vi "Channel Performance Lookup Test.vi"() -> ()   [LabVIEW 2021]
uses:
  <vilib>/Platform/TimedLoop/XDataNode/timing_clust.ctl
  <vilib>/Platform/TimedLoop/XDataNode/nitl_modes.ctl
  <vilib>/Platform/TimedLoop/XDataNode/wakeup.ctl
  <vilib>/Platform/TimedLoop/XDataNode/XDataNode.xnode
  <vilib>/Platform/TimedLoop/XDataNode/XDNodeRunTimeDep.lvlib
panel:
  out "Average Empty":dbl
  out "Max Empty":dbl
  out "Avg simple string":dbl
  out "Max simple varied string":dbl
  out "Avg simple i32":dbl
  out "Max simple i32":dbl
  out "Avg simple string":dbl
  out "Max simple string":dbl
  out "pass":bool
  # "This test should be run on RT.  It stresses the communications by constantly creating resource contraints with the low priority sender and the high priority loop. On Windows the priority of the loops cannot be set."
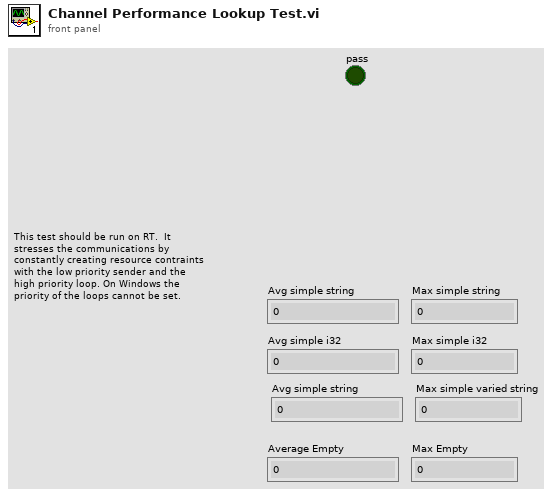
[diagram p1: front panel]
types:
  T1 = typedef "XDNodeRunTimeDep.lvlib/timing_clust.ctl" = cluster{"Expected End [f-1]":u64, "Actual End [f-1]":u64, "Finished Late? [f-1]":bool, "Expected End [i-1]":u64, "Actual End [i-1]":u64, "Finished Late? [i-1]":bool, "Expected Start [i]":u64, "Actual Start [i]":u64, "Expected Start [f]":u64, "Actual Start [f]":u64, "Source Name":string, "Structure Name":string, "Period":i64, "Deadline":i64, "Offset":i64, "Start":i64, "Priority":i32, "Timeout":i32, "Mode":T2, "Wakeup Reason":T3, "Error":errorcluster, "Source Type":string, "Secondary Source Type":string, "Global End Time":u64, "Global Start Time":u64, "Frame Duration":u64, "Iteration Duration":u64, "Assigned CPU":i32, "I/O Scan Engine Mode":u32}
  T2 = typedef "XDNodeRunTimeDep.lvlib/nitl_modes.ctl" = enum32{"No Change", "Process missed periods, maintain original phase", "Discard missed periods, maintain original phase", "Process missed periods, ignore original phase", "Discard missed periods, ignore original phase"}
  T3 = typedef "XDNodeRunTimeDep.lvlib/wakeup.ctl" = enum32{"Normal", "Aborted", "Asynchronous wakeup", "Timing source error", "Timed loop error", "Timeout"}
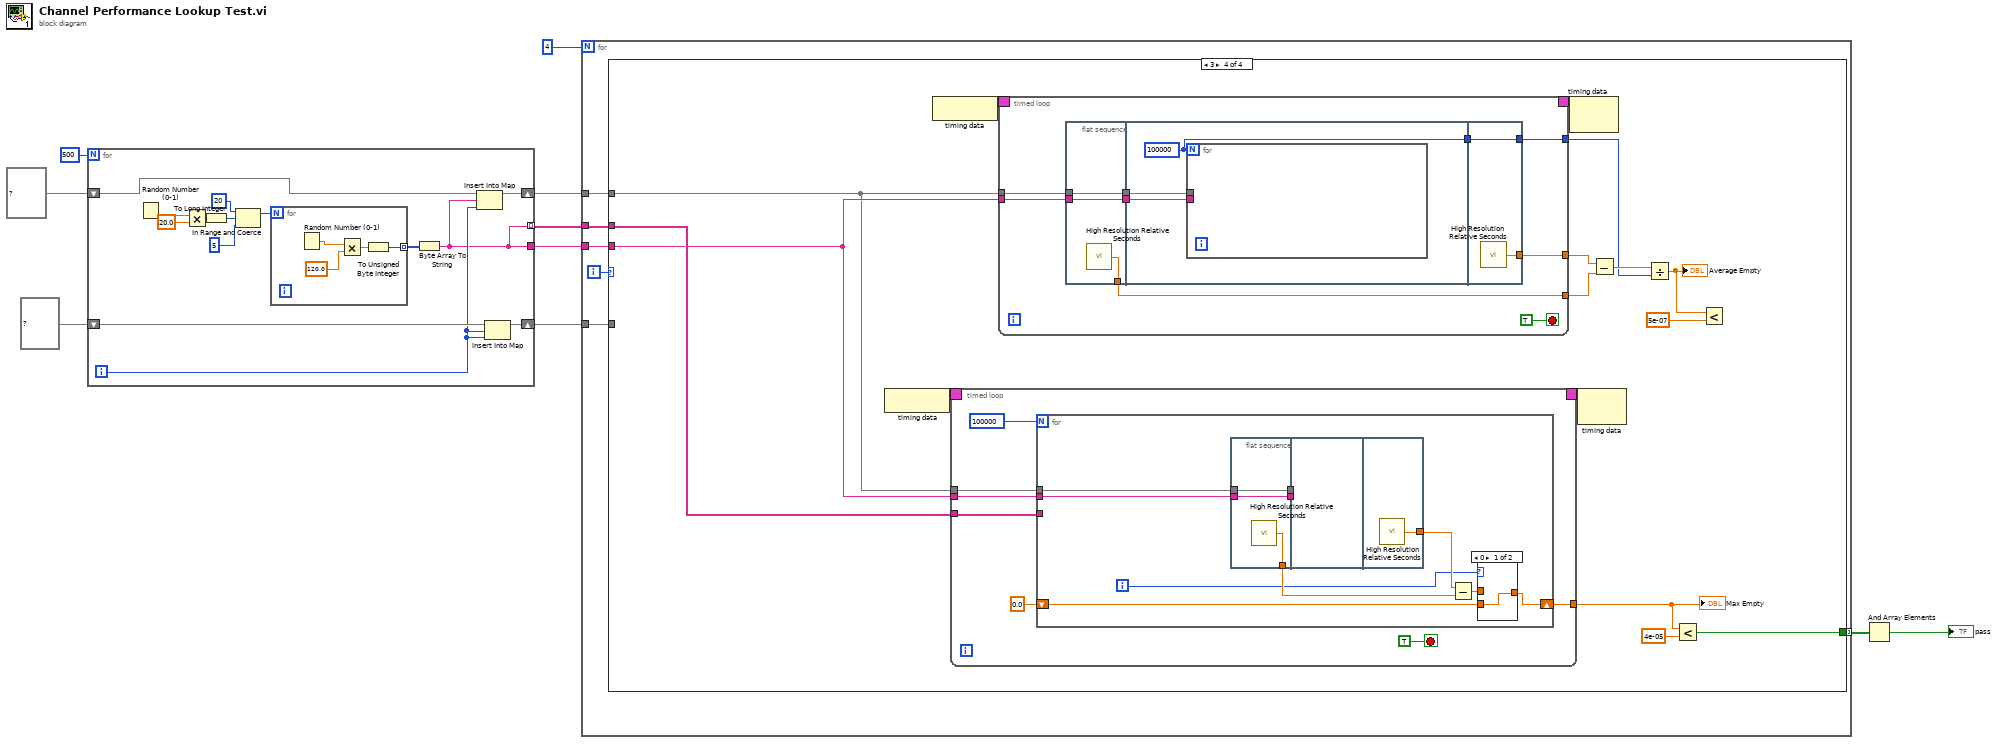
[diagram p0: block diagram]
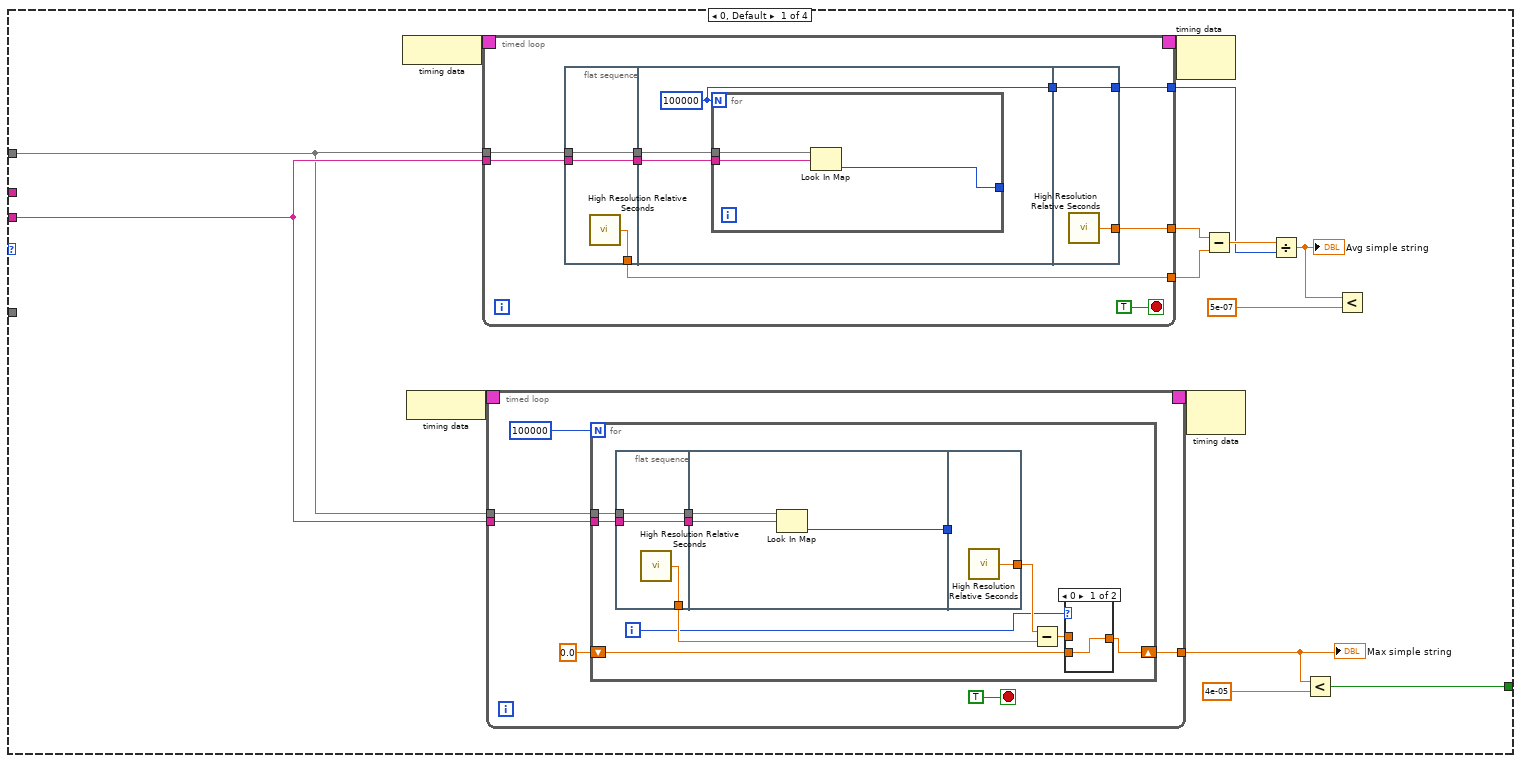
[diagram p2: hidden frame]
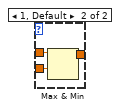
[diagram p3: hidden frame]
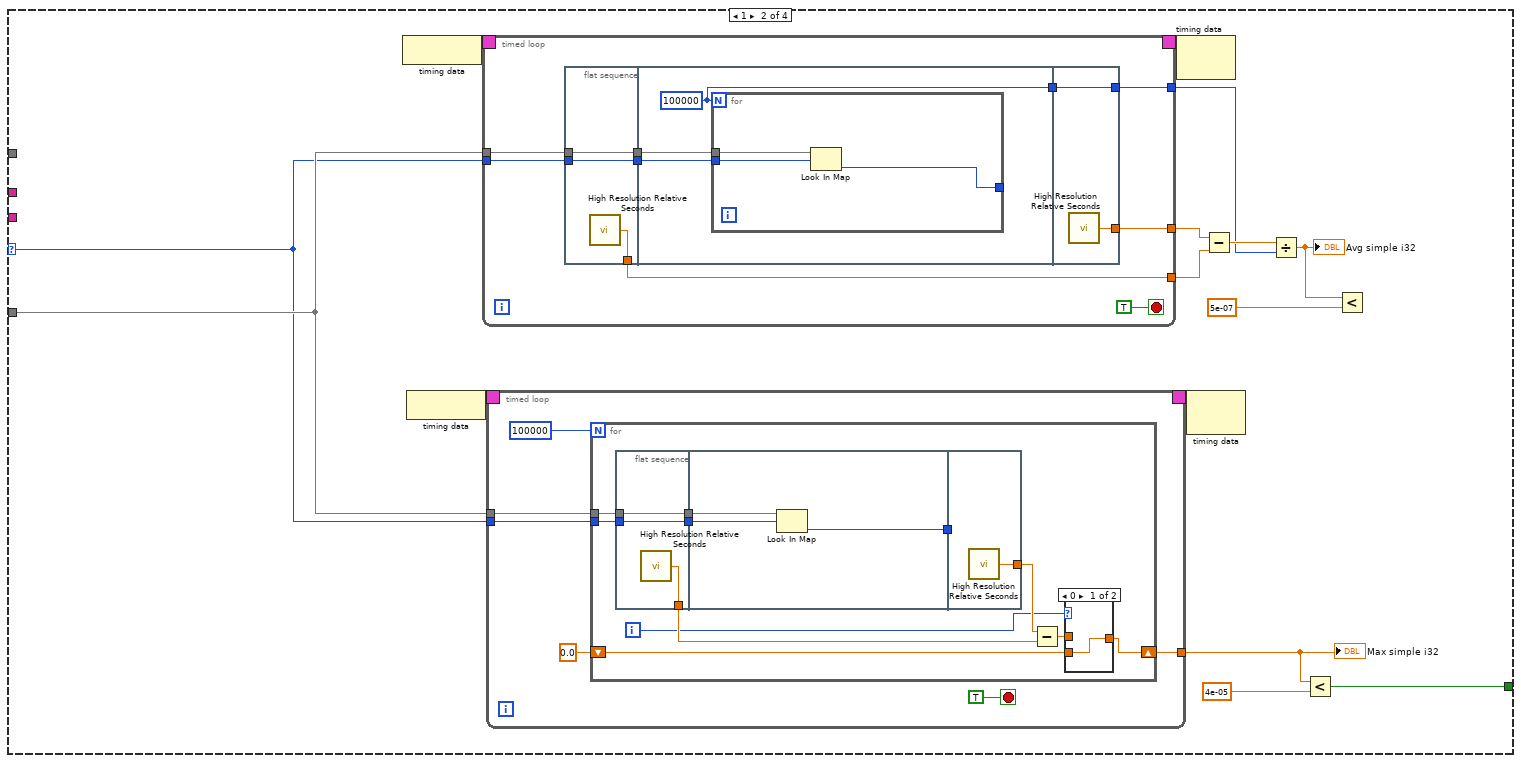
[diagram p4: hidden frame]
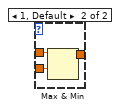
[diagram p5: hidden frame]
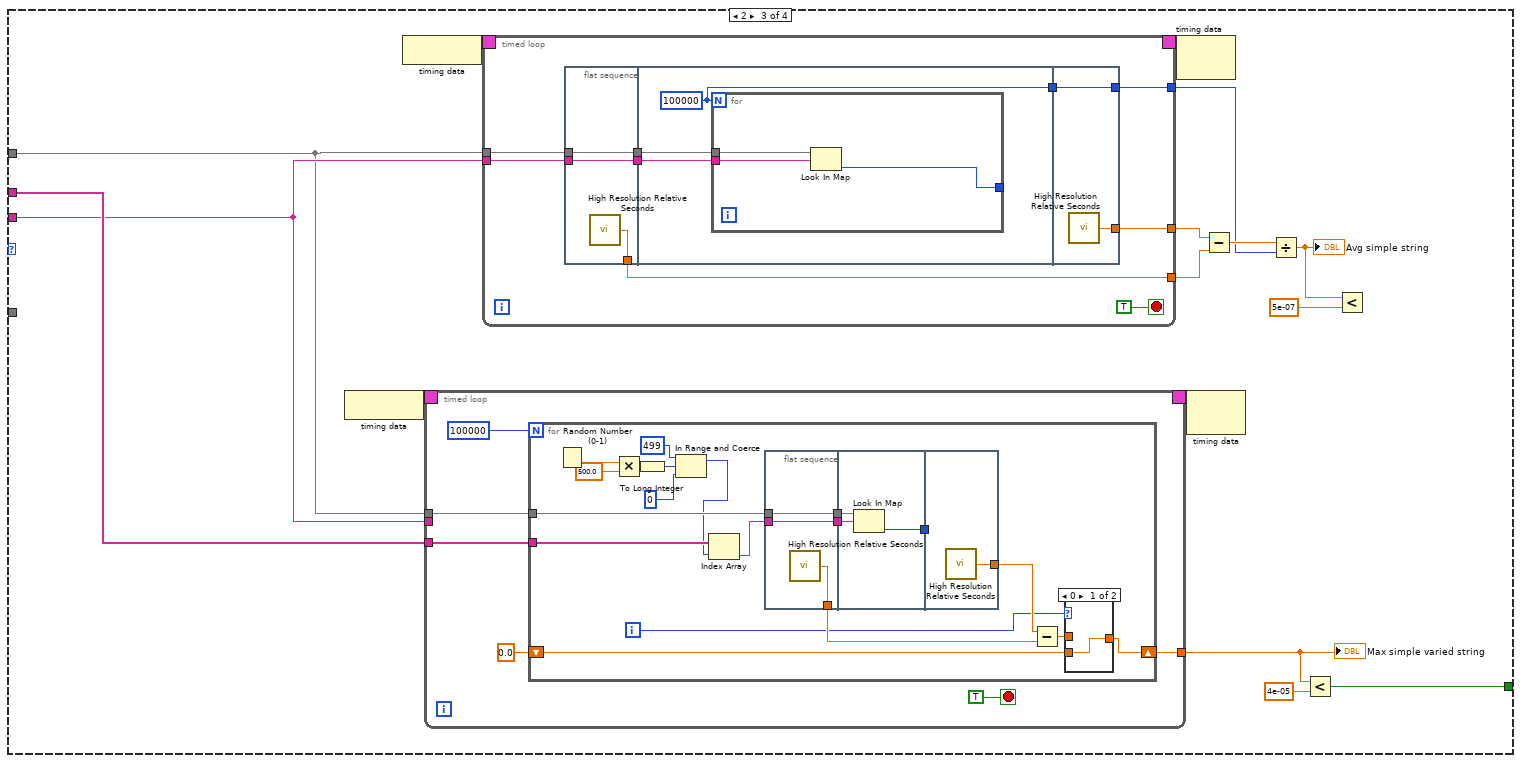
[diagram p6: hidden frame]
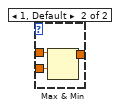
[diagram p7: hidden frame]
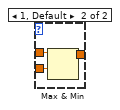
[diagram p8: hidden frame]
diagram:
  n1 = for {
    N: 500 -> [_]
    shift-right: [w16] -> w4
    shift-left: map{string, i32} {} ("map") -> [w15]
    tunnel: [w11] -> w3
    shift-right: [w13] -> w2
    shift-left: map{i32, i32} {} ("map") -> [w14]
    tunnel: [w11] -> w1 mode=indexing
    i -> [w12]
    n2 = Random Number (0-1)() -> (number: 0 to 1=w24:dbl)
    n3 = Multiply(x=w24, y=20.0) -> (x*y=w22:dbl)
    n4 = To Long Integer(number=w22) -> (32bit integer=w21:i32)
    n5 = In Range and Coerce(upper limit=20, x=w21, lower limit=5) -> (coerced(x)=w18:i32)  [unwired: 1 out]
    n6 = for {
      N: w18 -> [_]
      tunnel: [w25] -> w17 mode=indexing
      n7 = Random Number (0-1)() -> (number: 0 to 1=w28:dbl)
      n8 = Multiply(x=w28, y=120.0) -> (x*y=w26:dbl)
      n9 = To Unsigned Byte Integer(number=w26) -> (unsigned 8bit integer=w25:u8)
    }
    n10 = Byte Array To String(unsigned byte array=w17) -> (string=w11:string)
    n11 = Insert Into Map(map in=w15, key=w11, value=w12) -> (map out=w16:map{string, i32})  [unwired: 2 out]
    n12 = Insert Into Map(map in=w14, key=w12, value=w12) -> (map out=w13:map{i32, i32})  [unwired: 2 out]
  }
  n13 = for {
    N: 4 -> [_]
    tunnel: [w34] -> w9 mode=indexing
    tunnel: w4 -> [w32]
    tunnel: w3 -> [w31]
    tunnel: w2 -> [w30]
    tunnel: w1 -> [w29]
    i -> [w33]
    n14 = case shown="3" w33 {
      selector: w33 -> [_ w106 _ _]
      tunnel: [w37 w108 w180 w260] -> w34
      tunnel: w32 -> [w35 _ w177 w257]
      tunnel: w31 -> [w36 _ w178 w258]
      tunnel: w30 -> [_ w107 _ _]
      tunnel: w29 -> [_ _ w179 w259]
      frame 0, Default {
        n15 = node-c288() -> (w49:T1)
        n16 = node-c288() -> (w47:T1)
        n17 = timed-loop {
          timing: w49 -> [_]
          timing-out: [_] -> w48
          tunnel: w35 -> [w90]
          tunnel: [w87] -> w45
          tunnel: [w86] -> w44
          tunnel: [w85] -> w42
          tunnel: w36 -> [w83]
          stop <- TRUE stop-if-true
          n18 = flat-sequence {
            tunnel: w90 -> [w93]
            tunnel: [w93] -> w88
            tunnel: [w92] -> w86
            tunnel: w83 -> [w91]
            tunnel: [w91] -> w82
            tunnel: w88 -> [w96]
            tunnel: [w95] -> w84
            tunnel: w82 -> [w94]
            tunnel: [w101] -> w87
            tunnel: [w100] -> w85
            tunnel: w84 -> [w100]
            frame #0 {
              n19 = call <vilib>:"High Resolution Relative Seconds.vi"() -> ("relative seconds"=w92:dbl)
            }
            frame #1 {
              w95 = 100000
              n20 = for {
                N: w95 -> [_]
                tunnel: [w98] -> _
                tunnel: w94 -> [w97]
                tunnel: w96 -> [w99]
                n21 = Look In Map(map=w99, key=w97) -> (value=w98:i32)  [unwired: 1 in, 1 out]
              }
            }
            frame #2 {
              n22 = call <vilib>:"High Resolution Relative Seconds.vi"() -> ("relative seconds"=w101:dbl)
            }
          }
        }
        n23 = timed-loop {
          timing: w47 -> [_]
          timing-out: [_] -> w46
          tunnel: w35 -> [w51]
          tunnel: w36 -> [w50]
          tunnel: [w52] -> w39
          stop <- TRUE stop-if-true
          n24 = for {
            N: 100000 -> [_]
            shift-right: [w60] -> w52
            shift-left: 0.0 -> [w61]
            tunnel: w51 -> [w58]
            tunnel: w50 -> [w57]
            i -> [w59]
            n25 = flat-sequence {
              tunnel: [w72] -> w66
              tunnel: [w73] -> w63
              tunnel: [w71] -> w65
              tunnel: w58 -> [w72]
              tunnel: w57 -> [w71]
              tunnel: w66 -> [w76]
              tunnel: w65 -> [w75]
              tunnel: [w74] -> w56
              tunnel: [w77] -> w64
              tunnel: w56 -> [_]
              frame #0 {
                n26 = call <vilib>:"High Resolution Relative Seconds.vi"() -> ("relative seconds"=w73:dbl)
              }
              frame #1 {
                n27 = Look In Map(map=w76, key=w75) -> (value=w74:i32)  [unwired: 1 in, 1 out]
              }
              frame #2 {
                n28 = call <vilib>:"High Resolution Relative Seconds.vi"() -> ("relative seconds"=w77:dbl)
              }
            }
            n29 = Subtract(x=w64, y=w63) -> (x-y=w62:dbl)
            n30 = case shown="0" w59 {
              tunnel: w62 -> [_ w70]
              tunnel: w61 -> [w67 w69]
              tunnel: [w67 w68] -> w60
              frame 0 {
              }
              frame 1, Default {
                n31 = Max & Min(x=w70, y=w69) -> (max(x,y)=w68:dbl)  [unwired: 1 out]
              }
            }
          }
        }
        "Max simple string" <- w39
        n32 = node-c288(w48) -> ()  [unwired: 1 out]
        n33 = node-c288(w46) -> ()  [unwired: 1 out]
        n34 = Subtract(x=w45, y=w44) -> (x-y=w43:dbl)
        n35 = Divide(x=w43, y=w42) -> (x/y=w41:dbl)
        "Avg simple string" <- w41
        n36 = Less?(x=w39, y=4e-05) -> (x < y?=w37:bool)
        n37 = Less?(x=w41, y=5e-07) -> ()  [unwired: 1 out]
      }
      frame 1 {
        n38 = node-c288() -> (w120:T1)
        n39 = node-c288() -> (w118:T1)
        n40 = timed-loop {
          timing: w120 -> [_]
          timing-out: [_] -> w119
          tunnel: w107 -> [w161]
          tunnel: [w158] -> w116
          tunnel: [w157] -> w115
          tunnel: [w156] -> w113
          tunnel: w106 -> [w154]
          stop <- TRUE stop-if-true
          n41 = flat-sequence {
            tunnel: w161 -> [w164]
            tunnel: [w164] -> w159
            tunnel: [w163] -> w157
            tunnel: w154 -> [w162]
            tunnel: [w162] -> w153
            tunnel: w159 -> [w167]
            tunnel: [w166] -> w155
            tunnel: w153 -> [w165]
            tunnel: [w172] -> w158
            tunnel: [w171] -> w156
            tunnel: w155 -> [w171]
            frame #0 {
              n42 = call <vilib>:"High Resolution Relative Seconds.vi"() -> ("relative seconds"=w163:dbl)
            }
            frame #1 {
              w166 = 100000
              n43 = for {
                N: w166 -> [_]
                tunnel: [w169] -> _
                tunnel: w165 -> [w168]
                tunnel: w167 -> [w170]
                n44 = Look In Map(map=w170, key=w168) -> (value=w169:i32)  [unwired: 1 in, 1 out]
              }
            }
            frame #2 {
              n45 = call <vilib>:"High Resolution Relative Seconds.vi"() -> ("relative seconds"=w172:dbl)
            }
          }
        }
        n46 = timed-loop {
          timing: w118 -> [_]
          timing-out: [_] -> w117
          tunnel: w107 -> [w122]
          tunnel: w106 -> [w121]
          tunnel: [w123] -> w110
          stop <- TRUE stop-if-true
          n47 = for {
            N: 100000 -> [_]
            shift-right: [w131] -> w123
            shift-left: 0.0 -> [w132]
            tunnel: w122 -> [w129]
            tunnel: w121 -> [w128]
            i -> [w130]
            n48 = flat-sequence {
              tunnel: [w143] -> w137
              tunnel: [w144] -> w134
              tunnel: [w142] -> w136
              tunnel: w129 -> [w143]
              tunnel: w128 -> [w142]
              tunnel: w137 -> [w147]
              tunnel: w136 -> [w146]
              tunnel: [w145] -> w127
              tunnel: [w148] -> w135
              tunnel: w127 -> [_]
              frame #0 {
                n49 = call <vilib>:"High Resolution Relative Seconds.vi"() -> ("relative seconds"=w144:dbl)
              }
              frame #1 {
                n50 = Look In Map(map=w147, key=w146) -> (value=w145:i32)  [unwired: 1 in, 1 out]
              }
              frame #2 {
                n51 = call <vilib>:"High Resolution Relative Seconds.vi"() -> ("relative seconds"=w148:dbl)
              }
            }
            n52 = Subtract(x=w135, y=w134) -> (x-y=w133:dbl)
            n53 = case shown="0" w130 {
              tunnel: w133 -> [_ w141]
              tunnel: w132 -> [w138 w140]
              tunnel: [w138 w139] -> w131
              frame 0 {
              }
              frame 1, Default {
                n54 = Max & Min(x=w141, y=w140) -> (max(x,y)=w139:dbl)  [unwired: 1 out]
              }
            }
          }
        }
        "Max simple i32" <- w110
        n55 = node-c288(w119) -> ()  [unwired: 1 out]
        n56 = node-c288(w117) -> ()  [unwired: 1 out]
        n57 = Subtract(x=w116, y=w115) -> (x-y=w114:dbl)
        n58 = Divide(x=w114, y=w113) -> (x/y=w112:dbl)
        "Avg simple i32" <- w112
        n59 = Less?(x=w110, y=4e-05) -> (x < y?=w108:bool)
        n60 = Less?(x=w112, y=5e-07) -> ()  [unwired: 1 out]
      }
      frame 2 {
        n61 = node-c288() -> (w190:T1)
        n62 = node-c288() -> (w192:T1)
        n63 = timed-loop {
          timing: w190 -> [_]
          timing-out: [_] -> w189
          tunnel: w177 -> [w194]
          tunnel: w178 -> [_]
          tunnel: [w195] -> w182
          tunnel: w179 -> [w193]
          stop <- TRUE stop-if-true
          n64 = for {
            N: 100000 -> [_]
            shift-right: [w211] -> w195
            shift-left: 0.0 -> [w212]
            tunnel: w194 -> [w210]
            tunnel: w193 -> [w208]
            i -> [w207]
            n65 = Random Number (0-1)() -> (number: 0 to 1=w205:dbl)
            n66 = Multiply(x=w205, y=500.0) -> (x*y=w203:dbl)
            n67 = To Long Integer(number=w203) -> (32bit integer=w202:i32)
            n68 = In Range and Coerce(upper limit=499, x=w202, lower limit=0) -> (coerced(x)=w199:i32)  [unwired: 1 out]
            n69 = Index Array(array=w208, index=w199) -> (element=w206:string)
            n70 = flat-sequence {
              tunnel: [w223] -> w217
              tunnel: [w224] -> w214
              tunnel: [w222] -> w216
              tunnel: w210 -> [w223]
              tunnel: w206 -> [w222]
              tunnel: w217 -> [w227]
              tunnel: w216 -> [w226]
              tunnel: [w225] -> w209
              tunnel: [w228] -> w215
              tunnel: w209 -> [_]
              frame #0 {
                n71 = call <vilib>:"High Resolution Relative Seconds.vi"() -> ("relative seconds"=w224:dbl)
              }
              frame #1 {
                n72 = Look In Map(map=w227, key=w226) -> (value=w225:i32)  [unwired: 1 in, 1 out]
              }
              frame #2 {
                n73 = call <vilib>:"High Resolution Relative Seconds.vi"() -> ("relative seconds"=w228:dbl)
              }
            }
            n74 = Subtract(x=w215, y=w214) -> (x-y=w213:dbl)
            n75 = case shown="0" w207 {
              tunnel: w213 -> [_ w221]
              tunnel: w212 -> [w218 w220]
              tunnel: [w218 w219] -> w211
              frame 0 {
              }
              frame 1, Default {
                n76 = Max & Min(x=w221, y=w220) -> (max(x,y)=w219:dbl)  [unwired: 1 out]
              }
            }
          }
        }
        "Max simple varied string" <- w182
        n77 = timed-loop {
          timing: w192 -> [_]
          timing-out: [_] -> w191
          tunnel: w177 -> [w241]
          tunnel: [w238] -> w188
          tunnel: [w237] -> w187
          tunnel: [w236] -> w185
          tunnel: w178 -> [w234]
          stop <- TRUE stop-if-true
          n78 = flat-sequence {
            tunnel: w241 -> [w244]
            tunnel: [w244] -> w239
            tunnel: [w243] -> w237
            tunnel: w234 -> [w242]
            tunnel: [w242] -> w233
            tunnel: w239 -> [w247]
            tunnel: [w246] -> w235
            tunnel: w233 -> [w245]
            tunnel: [w252] -> w238
            tunnel: [w251] -> w236
            tunnel: w235 -> [w251]
            frame #0 {
              n79 = call <vilib>:"High Resolution Relative Seconds.vi"() -> ("relative seconds"=w243:dbl)
            }
            frame #1 {
              w246 = 100000
              n80 = for {
                N: w246 -> [_]
                tunnel: [w249] -> _
                tunnel: w245 -> [w248]
                tunnel: w247 -> [w250]
                n81 = Look In Map(map=w250, key=w248) -> (value=w249:i32)  [unwired: 1 in, 1 out]
              }
            }
            frame #2 {
              n82 = call <vilib>:"High Resolution Relative Seconds.vi"() -> ("relative seconds"=w252:dbl)
            }
          }
        }
        n83 = node-c288(w191) -> ()  [unwired: 1 out]
        n84 = node-c288(w189) -> ()  [unwired: 1 out]
        n85 = Subtract(x=w188, y=w187) -> (x-y=w186:dbl)
        n86 = Divide(x=w186, y=w185) -> (x/y=w184:dbl)
        "Avg simple string" <- w184
        n87 = Less?(x=w182, y=4e-05) -> (x < y?=w180:bool)
        n88 = Less?(x=w184, y=5e-07) -> ()  [unwired: 1 out]
      }
      frame 3 {
        n89 = node-c288() -> (w270:T1)
        n90 = node-c288() -> (w272:T1)
        n91 = timed-loop {
          timing: w270 -> [_]
          timing-out: [_] -> w269
          tunnel: w257 -> [w275]
          tunnel: w258 -> [w273]
          tunnel: [w276] -> w262
          tunnel: w259 -> [w274]
          stop <- TRUE stop-if-true
          n92 = for {
            N: 100000 -> [_]
            shift-right: [w285] -> w276
            shift-left: 0.0 -> [w286]
            tunnel: w275 -> [w282]
            tunnel: w274 -> [_]
            tunnel: w273 -> [w280]
            i -> [w284]
            n93 = flat-sequence {
              tunnel: [w296] -> w288
              tunnel: [w295] -> w283
              tunnel: w282 -> [w295]
              tunnel: [w294] -> w281
              tunnel: w280 -> [w294]
              tunnel: w283 -> [_]
              tunnel: w281 -> [_]
              tunnel: [w297] -> w289
              frame #0 {
                n94 = call <vilib>:"High Resolution Relative Seconds.vi"() -> ("relative seconds"=w296:dbl)
              }
              frame #1 {
              }
              frame #2 {
                n95 = call <vilib>:"High Resolution Relative Seconds.vi"() -> ("relative seconds"=w297:dbl)
              }
            }
            n96 = Subtract(x=w289, y=w288) -> (x-y=w287:dbl)
            n97 = case shown="0" w284 {
              tunnel: w287 -> [_ w293]
              tunnel: w286 -> [w290 w292]
              tunnel: [w290 w291] -> w285
              frame 0 {
              }
              frame 1, Default {
                n98 = Max & Min(x=w293, y=w292) -> (max(x,y)=w291:dbl)  [unwired: 1 out]
              }
            }
          }
        }
        "Max Empty" <- w262
        n99 = timed-loop {
          timing: w272 -> [_]
          timing-out: [_] -> w271
          tunnel: w257 -> [w310]
          tunnel: [w307] -> w268
          tunnel: [w306] -> w267
          tunnel: [w305] -> w265
          tunnel: w258 -> [w303]
          stop <- TRUE stop-if-true
          n100 = flat-sequence {
            tunnel: w310 -> [w313]
            tunnel: [w313] -> w308
            tunnel: [w312] -> w306
            tunnel: w303 -> [w311]
            tunnel: [w311] -> w302
            tunnel: w308 -> [w316]
            tunnel: [w315] -> w304
            tunnel: w302 -> [w314]
            tunnel: [w318] -> w307
            tunnel: [w317] -> w305
            tunnel: w304 -> [w317]
            frame #0 {
              n101 = call <vilib>:"High Resolution Relative Seconds.vi"() -> ("relative seconds"=w312:dbl)
            }
            frame #1 {
              w315 = 100000
              n102 = for {
                N: w315 -> [_]
                tunnel: w314 -> [_]
                tunnel: w316 -> [_]
              }
            }
            frame #2 {
              n103 = call <vilib>:"High Resolution Relative Seconds.vi"() -> ("relative seconds"=w318:dbl)
            }
          }
        }
        n104 = node-c288(w271) -> ()  [unwired: 1 out]
        n105 = node-c288(w269) -> ()  [unwired: 1 out]
        n106 = Subtract(x=w268, y=w267) -> (x-y=w266:dbl)
        n107 = Divide(x=w266, y=w265) -> (x/y=w264:dbl)
        "Average Empty" <- w264
        n108 = Less?(x=w262, y=4e-05) -> (x < y?=w260:bool)
        n109 = Less?(x=w264, y=5e-07) -> ()  [unwired: 1 out]
      }
    }
  }
  n110 = And Array Elements(Boolean array=w9) -> (logical AND=→"pass":bool)
